vi "MATLAB dtype string to Constant Variant.vi"(1 "Combo Box":string(combo)) -> (0 "Constant Variant":variant)   [LabVIEW 2018]
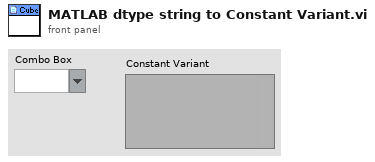
[diagram p1: front panel]
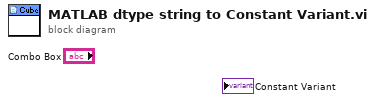
[diagram p0: block diagram]
diagram:
